vi "Merge.vi"(10 "Cache Managers":refnum<class "ConfigManager.Cache.lvclass">[](array[class])) -> (2 "Merged Cache":refnum<class "ConfigManager.Cache.lvclass">)   [LabVIEW 2013, in "SMOConfig.lvlib" / "ConfigManager.Cache.lvclass"]
uses:
  ConfigManager.Cache.lvclass
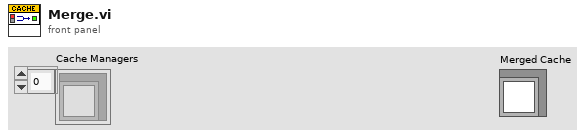
[diagram p1: front panel]
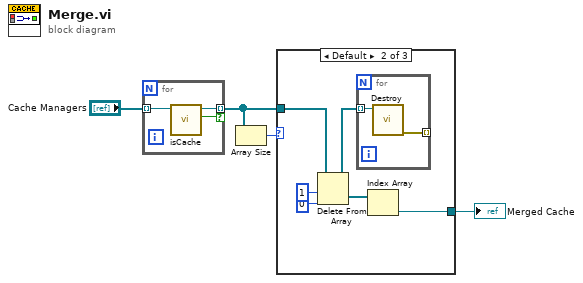
[diagram p0: block diagram]
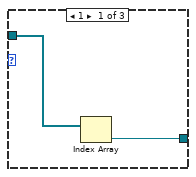
[diagram p2: hidden frame]
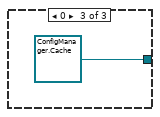
[diagram p3: hidden frame]
diagram:
  n1 = for {
    tunnel: "Cache Managers" -> [w7] mode=indexing
    tunnel: [w6] -> w3 mode=indexing if=w5
    n2 = call "isCache.vi"("ConfigManager.Cache in"=w7) -> ("isCache?"=w5:bool, "ConfigManager.Cache out"=w6:refnum<class "ConfigManager.Cache.lvclass">)  [unwired: 9 in]
  }
  n3 = Array Size(array=w3) -> (size(s)=w4:i32)
  n4 = case shown="Default" w4 {
    tunnel: w3 -> [w9 w15 _]
    tunnel: [w8 w11 refnum<class "ConfigManager.Cache.lvclass"> refnum ("Cache")] -> w1
    frame 1 {
      n5 = Index Array(array=w9) -> (element=w8:refnum<class "ConfigManager.Cache.lvclass">)  [unwired: 1 in]
    }
    frame Default {
      n6 = Delete From Array(array=w15, length=1, index=0) -> (deleted portion=w12:refnum<class "ConfigManager.Cache.lvclass">[], array with subset deleted=w10:refnum<class "ConfigManager.Cache.lvclass">[])
      n7 = for {
        tunnel: w10 -> [w17] mode=indexing
        tunnel: [w16] -> _ mode=indexing
        n8 = call-dynamic "Destroy.vi"("ConfigManager.Cache in"=w17) -> ("error out"=w16:errorcluster)  [unwired: 9 in, 1 out]
      }
      n9 = Index Array(array=w12) -> (element=w11:refnum<class "ConfigManager.Cache.lvclass">)  [unwired: 1 in]
    }
    frame 0 {
    }
  }
  "Merged Cache" <- w1
